vi "array up.vi"(8 "error in (no error)":errorcluster, 11 "Array in":refnum<vi>) -> (0 "error out":errorcluster, 3 "Array out":refnum<vi>)   [LabVIEW 2014, in "Tagbus PID Module editor node.lvclass"]
uses:
  Tagbus PID Module editor node.lvclass
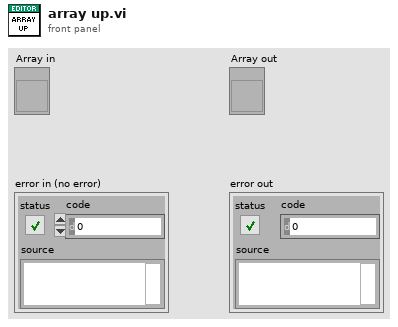
[diagram p1: front panel]
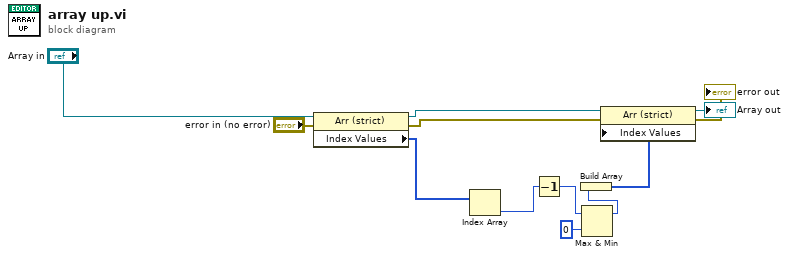
[diagram p0: block diagram]
diagram:
  n1 = property class="Arr (strict)"(reference="Array in", error in="error in (no error)") -> (reference out=w2:refnum<vi>, error out=w9:errorcluster, "Index Values"=w4:u32[])
  n2 = Index Array(array=w4) -> (element=w5:u32)  [unwired: 1 in]
  n3 = Decrement(x=w5) -> (x-1=w6:u32)
  n4 = Max & Min(x=w6, y=u32 0) -> (max(x,y)=w8:u32)  [unwired: 1 out]
  n5 = Build Array(w8) -> (w3:u32[])
  n6 = property class="Arr (strict)"(reference=w2, error in=w9, "Index Values"=w3) -> (reference out=→"Array out":refnum<vi>, error out=→"error out":errorcluster)
